vi "onRemoveHeader.vi"(8 "error in":errorcluster, 10 "header":string, 11 "REST Client in":refnum<class "REST Client.lvclass">) -> (0 "error out":errorcluster, 3 "REST Client out":refnum<class "REST Client.lvclass">)   [LabVIEW 2020, in "REST Client.lvlib" / "REST Client.lvclass"]
uses:
  REST Client.lvclass
  REST Client.lvclass/REST Client.ctl
  http-client-pkg/httpHeaders/httpHeaders.lvclass
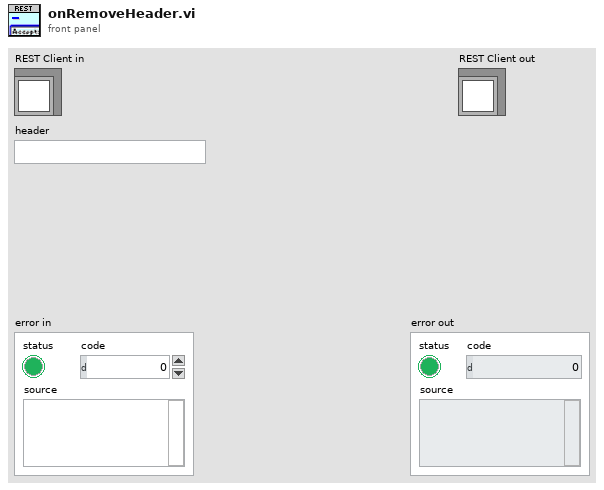
[diagram p1: front panel]
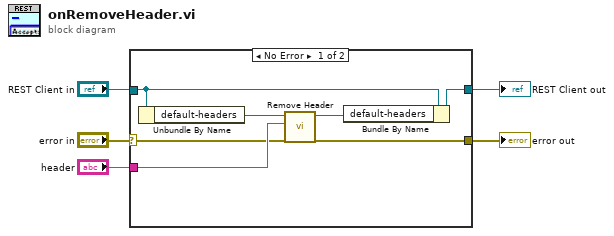
[diagram p0: block diagram]
diagram:
  n1 = case shown="No Error" "error in" {
    selector: "error in" -> [w7 w13]
    tunnel: "header" -> [w8 _]
    tunnel: "REST Client in" -> [w12 w14]
    tunnel: [w11 w14] -> w3
    tunnel: [w6 w13] -> w2
    frame No Error {
      n2 = Unbundle By Name(w12) -> ("default-headers"=w10:refnum<class "httpHeaders.lvclass">)
      n3 = call "Remove Header.vi"("error in (no error)"=w7, "header"=w8, "httpHeaders in"=w10) -> ("error out"=w6:errorcluster, "httpHeaders out"=w9:refnum<class "httpHeaders.lvclass">)  [unwired: 7 in]
      n4 = Bundle By Name(cluster=w12, "default-headers"=w9) -> (w11:refnum<class "REST Client.lvclass">)
    }
    frame Error {
    }
  }
  "error out" <- w2
  "REST Client out" <- w3
